vi "EnumToString.vi"(11 "Enum":variant) -> (3 "String":string)   [LabVIEW 2018]
uses:
  <vilib>/Utility/Data Type/NI_Data Type.lvlib
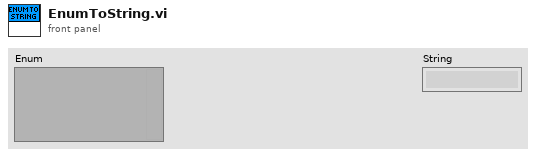
[diagram p1: front panel]
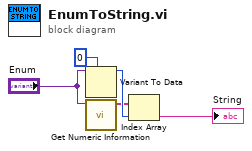
[diagram p0: block diagram]
diagram:
  n1 = Variant To Data(type=0, Variant="Enum") -> (data=w5:i32)  [unwired: 1 in, 1 out]
  n2 = call <vilib>:"Get Numeric Information.vi"("Variant"="Enum") -> ("Enum Names"=w4:string[])  [unwired: 7 in, 3 out]
  n3 = Index Array(array=w4, index=w5) -> (element=→"String":string)
